vi "generate fifo value.vi"(8 "data":u8, 9 "index":u8, 10 "device":u8, 11 "header":T1=enum."Input") -> (3 "Element":u32)   [LabVIEW 2013]
uses:
  profibus master transmit header.ctl
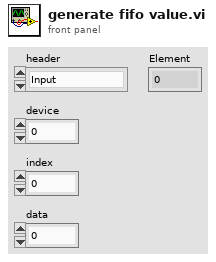
[diagram p1: front panel]
types:
  T1 = typedef "profibus master transmit header.ctl" = enum8{"Error", "Input", "Output", "Diagnostic", "input size", "output size"}
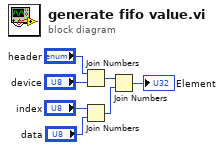
[diagram p0: block diagram]
diagram:
  n1 = Join Numbers(hi="header", lo="device") -> ((hi.lo)=w6:u16)
  n2 = Join Numbers(hi="index", lo="data") -> ((hi.lo)=w7:u16)
  n3 = Join Numbers(hi=w6, lo=w7) -> ((hi.lo)=→"Element":u32)
